vi "AlazarErrorToText.vi"(1 "Message":string, 2 "Error Code":u32) -> (0 "Text":string)   [LabVIEW 2018]
doc: "Convert a numerical return code to a NULL terminated string."
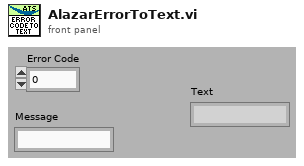
[diagram p1: front panel]
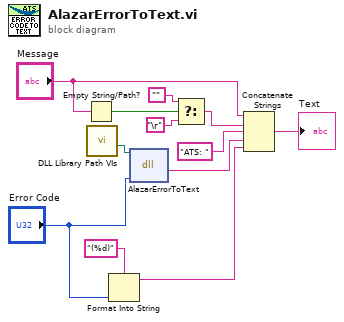
[diagram p0: block diagram]
diagram:
  n1 = Empty String/Path?(string/path="Message") -> (empty?=w4:bool)
  n2 = call "DLL Library Path VIs.vi"() -> ("Alazar"=w1:path)  [unwired: 9 in, 2 out]
  n3 = Format Into String(format string="(%d)", "Error Code") -> (resulting string=w8:string)  [unwired: 2 in, 1 out]
  n4 = dll-call lib="C:/Project/SerialSectOCT - FFT GPU/SerialSectOCT/Labview Software/DLL/ATSApi.dll" fn="AlazarErrorToText"(path in=w1, "ErrorCode"="Error Code") -> ("return type"=w7:string)  [unwired: 3 in, 2 out]
  n5 = Select(t="", s=w4, f="\r") -> (s? t:f=w10:string)
  n6 = Concatenate Strings("Message", w10, "ATS: ", w7, w8) -> (→"Text":string)
